vi "CAN Write.vi"(8 "error in (no error)":errorcluster caption="错误输入（无错误）", 10 "MessageBuffer":T1, 11 "Channel":u8) -> (0 "error out":errorcluster caption="错误输出", 2 "MessageBuffer out":T1, 3 "function return":u32)   [LabVIEW 2021]
doc: "TPCANStatus __stdcall CAN_Write(\n TPCANHandle Channel, \n TPCANMsg* MessageBuffer);"
uses:
  PCANBasic.dll
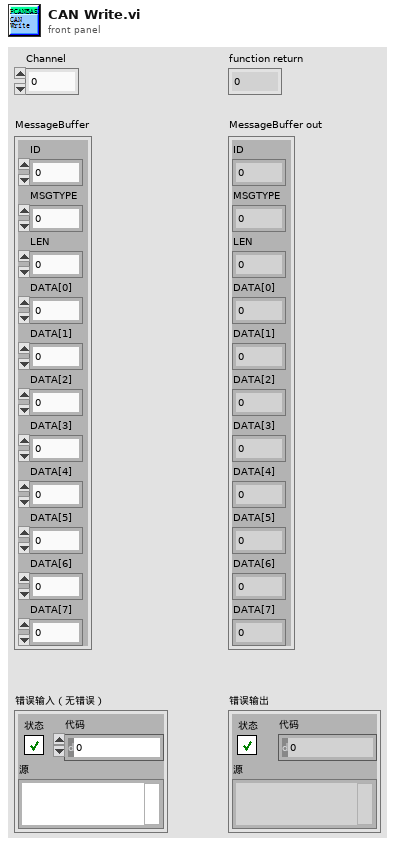
[diagram p1: front panel]
types:
  T1 = cluster{"ID":u32, "MSGTYPE":u8, "LEN":u8, "DATA[0]":u8, "DATA[1]":u8, "DATA[2]":u8, "DATA[3]":u8, "DATA[4]":u8, "DATA[5]":u8, "DATA[6]":u8, "DATA[7]":u8}
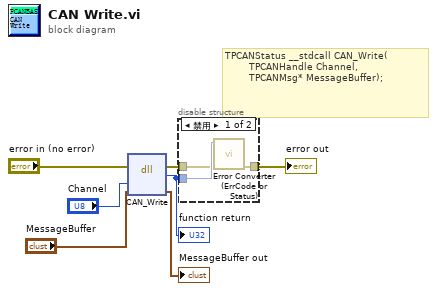
[diagram p0: block diagram]
diagram:
  # "TPCANStatus __stdcall CAN_Write(\n        TPCANHandle Channel, \n        TPCANMsg* MessageBuffer);"
  n1 = dll-call lib="D:/ON LINE WORK/LabVIEW/PCAN/PCAN 1.6(2021)/PCANBasic.dll" fn="CAN_Write"(error in="error in (no error)", "Channel"="Channel", "MessageBuffer"="MessageBuffer") -> (error out=w2:errorcluster, "返回类型"=w7:u32, "MessageBuffer"=→"MessageBuffer out":T1)  [unwired: 3 in, 1 out]
  "function return" <- w7
  n2 = disable-structure shown="禁用" {
    disable-tunnel: w7 -> [w10 _]
    disable-tunnel: w2 -> [w9 _]
    disable-tunnel: [w8 _] -> w1
    frame Disabled {
      n3 = call "Error Converter (ErrCode or Status).vi"("error in (no error)"=w9, "error code"=w10) -> ("error out"=w8:errorcluster)  [unwired: 9 in]
    }
    frame Enabled {
    }
  }
  "error out" <- w1
